vi "Query Result Name.vi"(8 "error IO":errorcluster, 11 "VISA resource name":refnum<visa-resource-name>) -> (0 "error Out":errorcluster, 2 "Result Name":string, 3 "VISA resource Out":refnum<visa-resource-name>)   [LabVIEW 2020, in "eec EST 300.lvlib"]
doc: "Query the Result Name setting."
uses:
  <instrlib>/eec EST 300/eec EST 300.lvlib
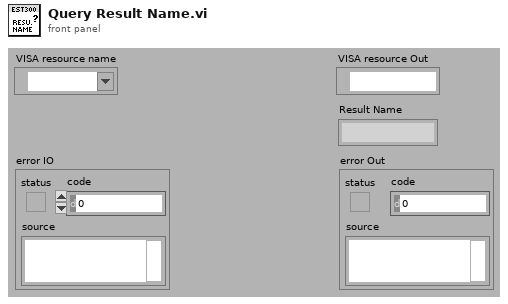
[diagram p1: front panel]
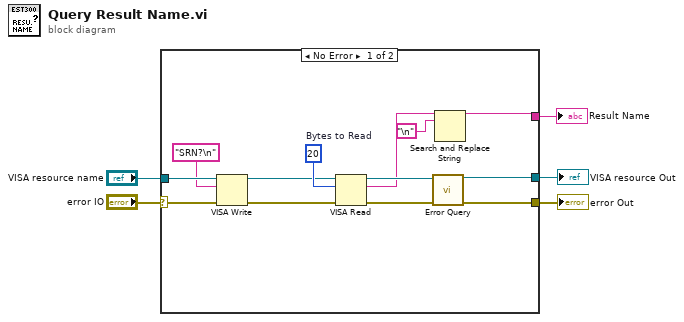
[diagram p0: block diagram]
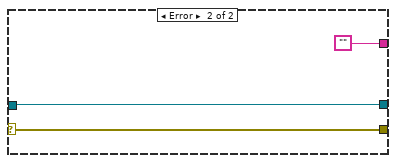
[diagram p2: hidden frame]
diagram:
  n1 = case shown="No Error" "error IO" {
    selector: "error IO" -> [w18 w21]
    tunnel: [w15 w21] -> w2
    tunnel: [w16 w20] -> w3
    tunnel: "VISA resource name" -> [w17 w20]
    tunnel: [w6 ""] -> w1
    frame No Error {
      w13 = u32 20  # Bytes to Read
      n2 = VISA Write(VISA resource name=w17, write buffer="SRN?\n" ("Command to Send (empty)"), error in (no error)=w18) -> (VISA resource name out=w10:refnum<visa-resource-name>, error out=w9:errorcluster)  [unwired: 1 out]
      n3 = VISA Read(VISA resource name=w10, byte count=w13, error in (no error)=w9) -> (VISA resource name out=w12:refnum<visa-resource-name>, read buffer=w8:string, error out=w11:errorcluster)  [unwired: 1 out]
      n4 = call <instrlib>:"Error Query.vi"("VISA resource name"=w12, "error in (no error)"=w11) -> ("VISA resource name out"=w16:refnum<visa-resource-name>, "error out"=w15:errorcluster)  [unwired: 10 in, 2 out]
      n5 = Search and Replace String(input string=w8, search string="\n") -> (result string=w6:string)  [unwired: 6 in, 3 out]
    }
    frame Error {
    }
  }
  "VISA resource Out" <- w3
  "error Out" <- w2
  "Result Name" <- w1
